vi "Auton-Initialize.vi"(8 "error in (no error)":errorcluster, 11 "Auton Methods":string[][](array[string])) -> (0 "error out":errorcluster, 3 "Auton Event Queue":refnum<queue>)   [LabVIEW 2014]
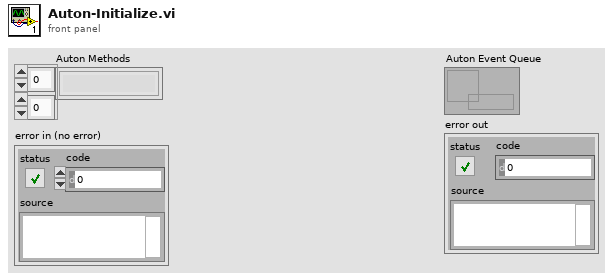
[diagram p1: front panel]
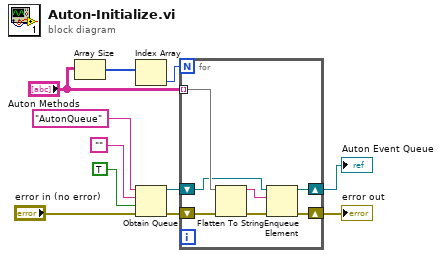
[diagram p0: block diagram]
diagram:
  n1 = Array Size(array="Auton Methods") -> (size(s)=w8:i32[])
  n2 = Index Array(array=w8) -> (element=w7:i32)  [unwired: 1 in]
  n3 = Obtain Queue(name (unnamed)="AutonQueue", element data type="", create if not found? (T)=TRUE, error in (no error)="error in (no error)") -> (queue out=w4:refnum<queue>, error out=w5:errorcluster)  [unwired: 1 in, 1 out]
  n4 = for {
    N: w7 -> [_]
    tunnel: "Auton Methods" -> [w18] mode=indexing
    shift-right: [w15] -> w2
    shift-left: w4 -> [w17]
    shift-right: [w12] -> w1
    shift-left: w5 -> [w14]
    n5 = Flatten To String(anything=w18, error in (no error)=w14) -> (data string=w16:string, error out=w13:errorcluster)  [unwired: 2 in, 1 out]
    n6 = Enqueue Element(queue=w17, element=w16, error in (no error)=w13) -> (queue out=w15:refnum<queue>, error out=w12:errorcluster)  [unwired: 1 in, 1 out]
  }
  "Auton Event Queue" <- w2
  "error out" <- w1
